vi "CreatePrivateEvents.vi"(8 "error in (no error)":errorcluster, 11 "DAQmx":refnum<class "DAQmx.lvclass">) -> (0 "error out":errorcluster, 3 "DAQmx out":refnum<class "DAQmx.lvclass">)   [LabVIEW 2019, in "DAQmx.lvclass"]
uses:
  DAQmx.lvclass
  typedefs/DAQ.Config.AO--Cluster--Array.ctl
  typedefs/DAQ.Config.AO--Cluster.ctl
  typedefs/DAQ.Config.AO.Range--enum.ctl
  typedefs/DAQ.Config.Device Type--enum.ctl
  typedefs/DAQ.Config.AI--Cluster--Array.ctl
  typedefs/DAQ.Config.AI--Cluster.ctl
  typedefs/DAQ.Config.AI.Coupling--enum.ctl
  typedefs/DAQ.Config.AI.Range--enum.ctl
  typedefs/DAQ.Config.Timing--Cluster.ctl
  typedefs/DAQ.Config.Timing.Sampling--Cluster.ctl
  typedefs/DAQ.Config.Timing.Fs Mode--enum.ctl
  typedefs/DAQmx.States--enum.ctl
  DAQmx.lvclass/DAQmx.ctl
  <vilib>/JKI/JKI SMO/SMO/SMO.lvclass
panel:
  # "For instructions on how to use the JKI State Machine Objects, examples and video tutorials, visit:\nhttp://jki.net/state-machine-objects/\n\nJKI State Machine Objects™\nhttp://jki.net/state-machine-objects/\nCopyright (C) 2005-2015, JKI <info@jki.net>\nALL RIGHTS RESERVED"
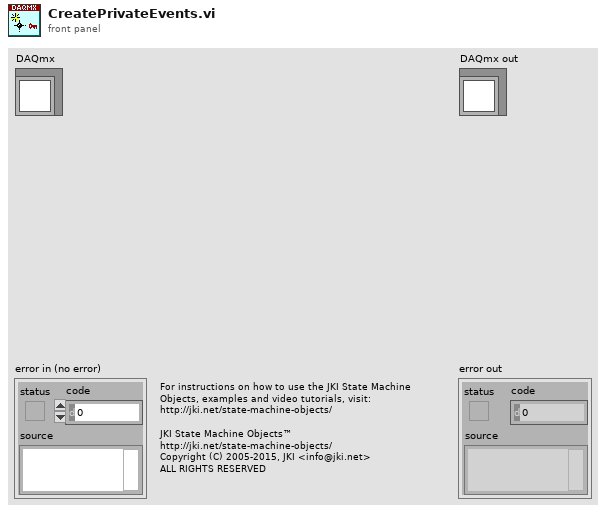
[diagram p1: front panel]
types:
  T1 = typedef "DAQmx.lvclass/DAQmx.States--enum.ctl" = enum16{"idle", "start", "stop", "calibrate", "auto"}
  T2 = typedef "DAQmx.lvclass/DAQ.Config.Timing--Cluster.ctl" = cluster{"Sampling":T3, "sample mode":i32, "FsMode":T4, "Fs Multiplier":dbl, "Refresh Rate (Hz)":dbl, "Decimation.PreDSP":i32, "Decimation.PostDSP":i32, "Fs.Output":dbl}
  T3 = typedef "DAQmx.lvclass/DAQ.Config.Timing.Sampling--Cluster.ctl" = cluster{"Fs":dbl, "#s":i32}
  T4 = typedef "DAQmx.lvclass/DAQ.Config.Timing.Fs Mode--enum.ctl" = enum16{"Manual", "Auto Fs", "Max Fs"}
  T5 = typedef "DAQmx.lvclass/DAQ.Config.AI--Cluster--Array.ctl" = T6[]
  T6 = typedef "DAQmx.lvclass/DAQ.Config.AI--Cluster.ctl" = cluster{"Channels":tag, "Coupling":T7, "Range":T8, "input terminal configuration":i32, "Type":T9}
  T7 = typedef "DAQmx.lvclass/DAQ.Config.AI.Coupling--enum.ctl" = u16
  T8 = typedef "DAQmx.lvclass/DAQ.Config.AI.Range--enum.ctl" = enum16{"±0.316", "±1.00", "±3.16", "±10.0", "±31.6", "±42.4", ""}
  T9 = typedef "DAQmx.lvclass/DAQ.Config.Device Type--enum.ctl" = enum16{"None", "USB-4431", "PXI-446x"}
  T10 = typedef "DAQmx.lvclass/DAQ.Config.AO--Cluster--Array.ctl" = T11[]
  T11 = typedef "DAQmx.lvclass/DAQ.Config.AO--Cluster.ctl" = cluster{"Channels":tag, "Range":T12, "output terminal configuration":i32, "Type":T9}
  T12 = typedef "DAQmx.lvclass/DAQ.Config.AO.Range--enum.ctl" = enum16{"±0.1", "±1.0", "±10.0", ""}
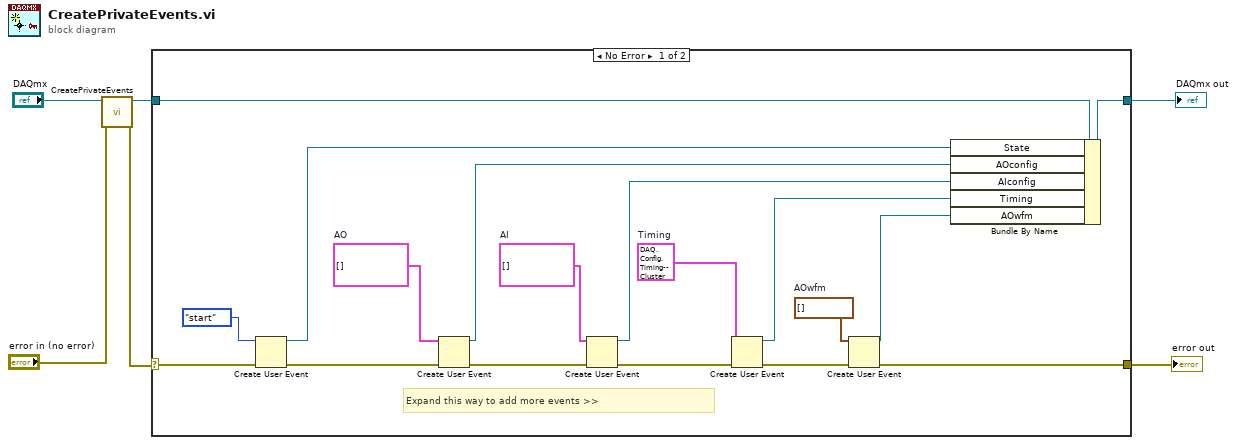
[diagram p0: block diagram]
diagram:
  n1 = call-parent "CreatePrivateEvents.vi"("error in (no error)"="error in (no error)", "SMO"="DAQmx") -> ("error out"=w4:errorcluster, "SMO out"=w5:refnum<class "DAQmx.lvclass">)  [unwired: 8 in]
  n2 = case shown="No Error" w4 {
    selector: w4 -> [w17 w26]
    tunnel: [w8 w26] -> w2
    tunnel: [w23 w25] -> w3
    tunnel: w5 -> [w24 w25]
    frame No Error {
      w11 = waveform(dbl)[] []  # AOwfm
      w7 = T2 {"Sampling"={"Fs"=1000.0, "#s"=128}, "sample mode"=10123, "FsMode"=enum."Manual", "Fs Multiplier"=1.0, "Refresh Rate (Hz)"=10.0, "Decimation.PreDSP"=1, "Decimation.PostDSP"=1, "Fs.Output"=204789.0}  # Timing
      w21 = T5 []  # AI
      w22 = T10 []  # AO
      # "Expand this way to add more events >>"
      n3 = Create User Event(user event datatype=DAQmx.States--enum."start" ("setState"), error in=w17) -> (user event=w15:refnum<user-event>, error out=w16:errorcluster)
      n4 = Create User Event(user event datatype=w22, error in=w16) -> (user event=w14:refnum<user-event>, error out=w20:errorcluster)
      n5 = Create User Event(user event datatype=w21, error in=w20) -> (user event=w13:refnum<user-event>, error out=w19:errorcluster)
      n6 = Create User Event(user event datatype=w7, error in=w19) -> (user event=w12:refnum<user-event>, error out=w10:errorcluster)
      n7 = Create User Event(user event datatype=w11, error in=w10) -> (user event=w9:refnum<user-event>, error out=w8:errorcluster)
      n8 = Bundle By Name(cluster=w24, "State"=w15, "AOconfig"=w14, "AIconfig"=w13, "Timing"=w12, "AOwfm"=w9) -> (w23:refnum<class "DAQmx.lvclass">)
    }
    frame Error {
    }
  }
  "error out" <- w2
  "DAQmx out" <- w3
